vi "Write Speed.vi"(8 "error in (no error)":errorcluster, 10 "Speed":dbl, 11 "MovementInstruction in":refnum<class "MovementInstruction.lvclass">) -> (0 "error out":errorcluster, 3 "MovementInstruction out":refnum<class "MovementInstruction.lvclass">)   [LabVIEW 2015, in "MovementInstruction.lvclass"]
uses:
  MovementInstruction.lvclass
  MovementInstruction.lvclass/MovementInstruction.ctl
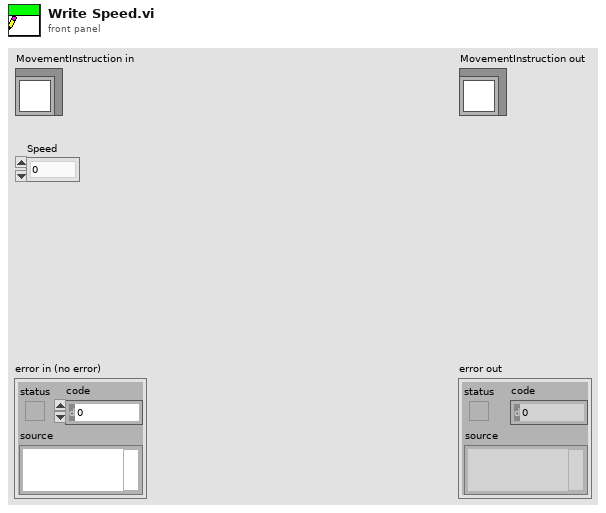
[diagram p1: front panel]
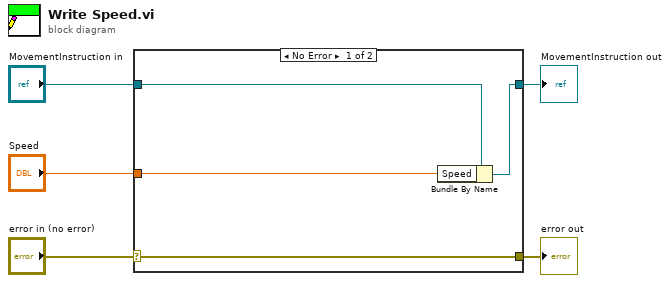
[diagram p0: block diagram]
diagram:
  n1 = case shown="No Error" "error in (no error)" {
    selector: "error in (no error)" -> [w9 w10]
    tunnel: [w9 w10] -> w4
    tunnel: [w7 w11] -> w2
    tunnel: "MovementInstruction in" -> [w8 w11]
    tunnel: "Speed" -> [w6 _]
    frame No Error {
      n2 = Bundle By Name(cluster=w8, "Speed"=w6) -> (w7:refnum<class "MovementInstruction.lvclass">)
    }
    frame Error {
    }
  }
  "error out" <- w4
  "MovementInstruction out" <- w2
